vi "Replace Brackets.vi"(4 "Label.Text":string) -> (1 "String":string)   [LabVIEW 2020]
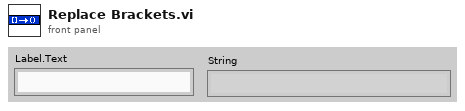
[diagram p1: front panel]
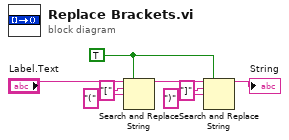
[diagram p0: block diagram]
diagram:
  w1 = TRUE ("replace all? (F)")
  n1 = Search and Replace String(replace all?=w1, input string="Label.Text", search string="[", replace string="(" ("replace string (\"\")")) -> (result string=w3:string)  [unwired: 1 in, 6 out]
  n2 = Search and Replace String(replace all?=w1, input string=w3, search string="]", replace string=")" ("replace string (\"\")")) -> (result string=→"String":string)  [unwired: 1 in, 6 out]
